vi "Save.vi"(8 "error in (no error)":errorcluster) -> (0 "error out":errorcluster)   [LabVIEW 2021, in "System Config.lvclass"]
uses:
  System Config.lvclass
  System Config.lvclass/System Config.ctl
  <vilib>/Utility/config.llb/NI_LVConfig.lvlib
  <userlib>/_OpenG.lib/variantconfig/variantconfig.llb/openg_variant_configuration_file.lvlib
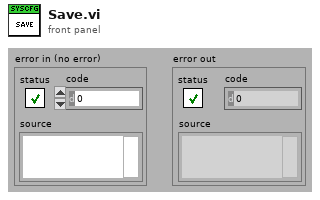
[diagram p1: front panel]
types:
  T1 = typedef "System Config.lvclass/ClassAttributesRef.ctl" = refnum<data-value>
  T2 = typedef "System Config.lvclass/ClassAttributes.ctl" = cluster{"Config":cluster{"Logging":cluster{"Log Files Directory":path, "Max Lines Per Log File":i32}, "Settings":T3}, "Core":cluster{"Config Directory":path, "Name":string, "Config Changed":refnum<user-event>}}
  T3 = typedef "System Config.lvclass/Settings.ctl" = cluster{"Dummy":dbl}
  T4 = cluster{"Logging":cluster{"Log Files Directory":path, "Max Lines Per Log File":i32}, "Settings":T3}
  T5 = typedef "NI_LVConfig.lvlib/Config Data RefNum.ctl" = refnum<k1>
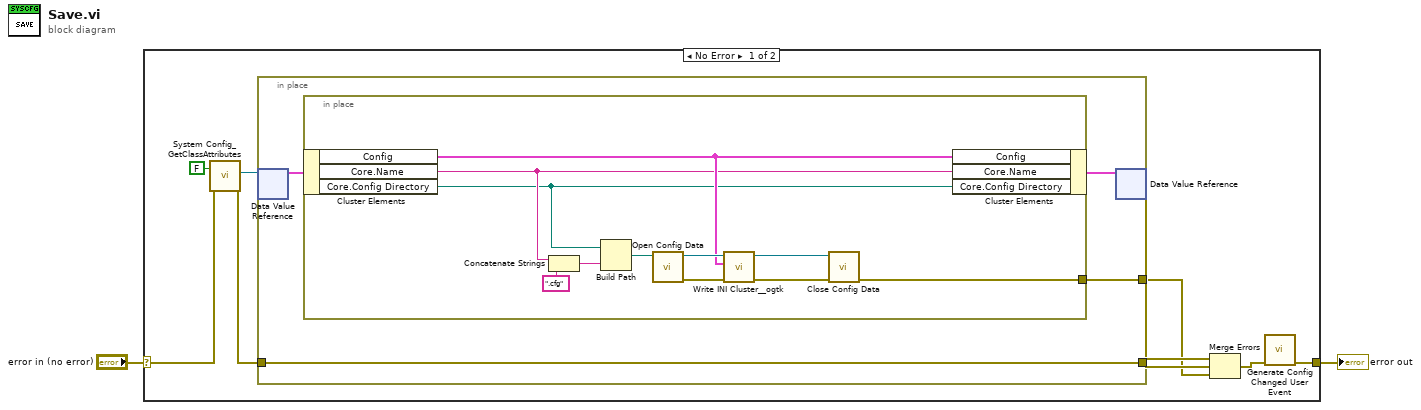
[diagram p0: block diagram]
diagram:
  n1 = case shown="No Error" "error in (no error)" {
    selector: "error in (no error)" -> [w11 w27]
    tunnel: [w4 w27] -> w1
    frame No Error {
      n2 = call "System Config_GetClassAttributes.vi"("error in (no error)"=w11, "return data? (T)"=FALSE ("return data")) -> ("error out"=w10:errorcluster, "class attributes ref"=w9:T1)  [unwired: 6 in, 2 out]
      n3 = in-place {
        in-place-border: w10 -> [w13]
        in-place-border: [w13] -> w7
        in-place-border: [w12] -> w3
        n4 = in-place-dvr #1(w9) -> (w14:T2)  [unwired: 1 out]
        n5 = in-place {
          in-place-border: [w19] -> w12
          n6 = in-place-cluster #2(w14) -> ("Config"=w18:T4, "Core.Name"=w17:string, "Core.Config Directory"=w16:path)
          n7 = Concatenate Strings(w17, ".cfg" ("string")) -> (w25:string)
          n8 = Build Path(base path=w16, name or relative path=w25) -> (appended path=w24:path)
          n9 = call <vilib>:"Open Config Data.vi"("configuration file path"=w24) -> ("error out"=w21:errorcluster, "refnum"=w23:T5)  [unwired: 8 in, 1 out]
          n10 = call <userlib>:"Write INI Cluster__ogtk.vi"("error in (no error)"=w21, "INI Fomatted Cluster"=w18, "refnum"=w23) -> ("error out"=w20:errorcluster, "dup refnum"=w22:T5)  [unwired: 7 in]
          n11 = call <vilib>:"Close Config Data.vi"("error in (no error)"=w20, "refnum"=w22) -> ("error out"=w19:errorcluster)  [unwired: 8 in, 1 out]
          n12 = in-place-cluster #2("Config"=w18, "Core.Name"=w17, "Core.Config Directory"=w16) -> (w15:T2)
        }
        n13 = in-place-dvr #1(w15) -> (w6:errorcluster)  [unwired: 1 out]
      }
      n14 = Merge Errors(w7, w6, w3) -> (w5:errorcluster)
      n15 = call "Generate Config Changed User Event.vi"("error in (no error)"=w5) -> ("error out"=w4:errorcluster)  [unwired: 10 in]
    }
    frame Error {
    }
  }
  "error out" <- w1
